vi "Set Operating Mode.vi"(8 "error in (no error)":errorcluster, 10 "Operating mode (0: Weighting)":u16(ring) items=["Weighing", "Parts Counting", "Deviations", "Dosing", "Formulas", "Animals Weighing", "Density", "Density of Solid Bodies", "Density of Liquids", "Peak Hold", "Totalizing", "Checkweighin", "Statistics", "Pipettes Calibration", "Differential Weighing", "Statistical Quality Control (SQC)", "Product Inspection", "Weight Control (Tableting)", "Drying", "Comparator", "Weighbridge"], 11 "VISA resource name":refnum<visa-resource-name>) -> (0 "error out":errorcluster, 3 "VISA resource name out":refnum<visa-resource-name>)   [LabVIEW 2017, in "RadWag balances and scales.lvlib"]
doc: "Setr balance in desired operating mode. Supported work modes can be checked with \"Get Available Operating Mode\" VI."
uses:
  <instrlib>/Prev/RadWag Continuous Read Folder/RadWag balances and scales.lvlib
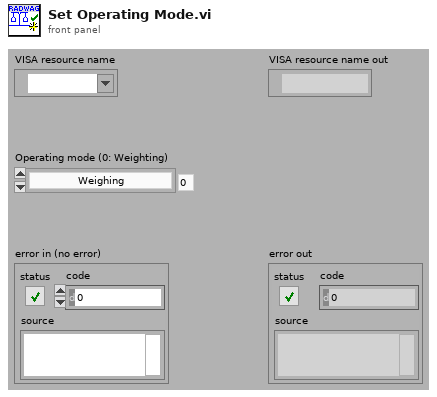
[diagram p1: front panel]
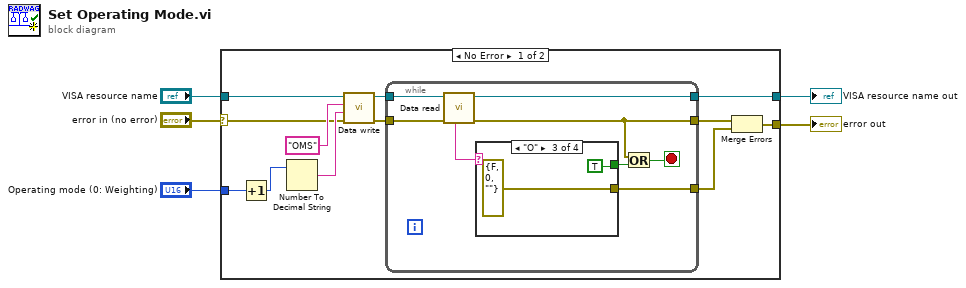
[diagram p0: block diagram]
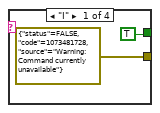
[diagram p2: hidden frame]
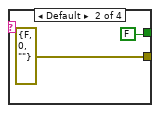
[diagram p3: hidden frame]
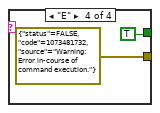
[diagram p4: hidden frame]
diagram:
  n1 = case shown="No Error" "error in (no error)" {
    selector: "error in (no error)" -> [w6 w34]
    tunnel: "Operating mode (0: Weighting)" -> [w14 _]
    tunnel: "VISA resource name" -> [w11 w35]
    tunnel: [w10 w35] -> w3
    tunnel: [w7 w34] -> w2
    frame No Error {
      n2 = Increment(x=w14) -> (x+1=w13:u16)
      n3 = Number To Decimal String(number=w13) -> (decimal integer string=w12:string)  [unwired: 1 in]
      n4 = call <instrlib>:"Data write.vi"("error in (no error)"=w6, "Parameter"=w12, "ID"="OMS", "VISA resource name"=w11) -> ("error out"=w16:errorcluster, "VISA resource name out"=w17:refnum<visa-resource-name>)  [unwired: 6 in]
      n5 = while {
        tunnel: w17 -> [w25]
        tunnel: w16 -> [w24]
        tunnel: [w20] -> w8
        tunnel: [w23] -> w10
        tunnel: [w22] -> w9
        stop <- w19 stop-if-true
        n6 = call <instrlib>:"Data read.vi"("error in (no error)"=w24, "VISA resource name"=w25) -> ("error out"=w20:errorcluster, "VISA resource name out"=w23:refnum<visa-resource-name>, "Status"=w18:string)  [unwired: 3 in, 4 out]
        n7 = case shown="\"O\"" w18 {
          tunnel: [errorcluster {"status"=FALSE, "code"=1073481728, "source"="Warning: Command currently unavailable"} ("t") errorcluster {"status"=FALSE, "code"=0, "source"=""} ("error constant") errorcluster {"status"=FALSE, "code"=0, "source"=""} ("error constant") errorcluster {"status"=FALSE, "code"=1073481732, "source"="Warning: Error in-course of command execution."} ("t")] -> w22
          tunnel: [TRUE FALSE TRUE TRUE] -> w21
          frame "I" {
          }
          frame Default {
          }
          frame "O" {
          }
          frame "E" {
          }
        }
        n8 = Or(x=w20, y=w21) -> (x .or. y?=w19:bool)
      }
      n9 = Merge Errors(w8, w9) -> (w7:errorcluster)
    }
    frame Error {
    }
  }
  "error out" <- w2
  "VISA resource name out" <- w3
